vi "Stop case cleanup.vi"(11 "Next State":T1) -> ()   [LabVIEW 2013]
uses:
  Typedefs/Top level VI states.ctl
  Typedefs/Next state queue data.ctl
  Typedefs/Start-Stop Enum.ctl
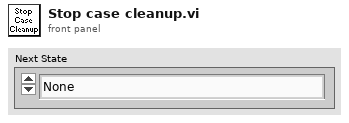
[diagram p1: front panel]
types:
  T1 = typedef "Top level VI states.ctl" = enum16{"None", "Initialise UI", "<STACK PROTOCOL STATES>", "AOL Zstack-START", "AOL Zstack-STOP", "Motor Zstack-START", "Motor Zstack-STOP", "<ACQUISITION PROTOCOL STATES> ", "Functional Acquisition-START", "Functional Acquisition-STOP", "Single Plane Acquisition-START", "Single Plane Acquisition-STOP", "Volume Acquisition-START", "Volume Acquisition-STOP", "<LIVE IMAGING PROTOCOL STATES>", "Live Imaging-START", "Live Imaging-STOP", "Live Plane Imaging-START", "Live Plane Imaging-STOP", "Live Volume Imaging-START", "Live Volume Imaging-STOP", "EXIT"}
  T2 = typedef "Start-Stop Enum.ctl" = enum16{"START", "STOP"}
  T3 = typedef "Next state queue data.ctl" = cluster{"Start/Stop":T2, "State":T1}
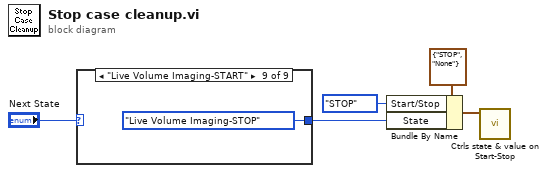
[diagram p0: block diagram]
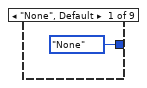
[diagram p2: hidden frame]
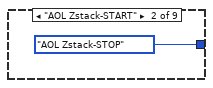
[diagram p3: hidden frame]
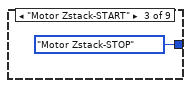
[diagram p4: hidden frame]
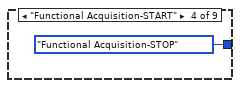
[diagram p5: hidden frame]
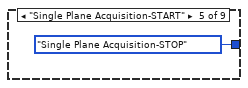
[diagram p6: hidden frame]
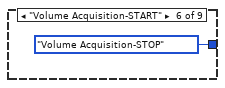
[diagram p7: hidden frame]
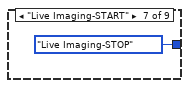
[diagram p8: hidden frame]
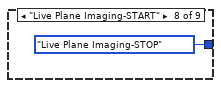
[diagram p9: hidden frame]
diagram:
  n1 = case shown="\"Live Volume Imaging-START\"" "Next State" {
    tunnel: [Top_level_VI_states."None" ("State") Top_level_VI_states."AOL Zstack-STOP" ("State") Top_level_VI_states."Motor Zstack-STOP" ("State") Top_level_VI_states."Functional Acquisition-STOP" ("State") Top_level_VI_states."Single Plane Acquisition-STOP" ("State") Top_level_VI_states."Volume Acquisition-STOP" ("State") Top_level_VI_states."Live Imaging-STOP" ("State") Top_level_VI_states."Live Plane Imaging-STOP" ("State") Top_level_VI_states."Live Volume Imaging-STOP" ("State")] -> w5
    frame "None", Default {
    }
    frame "AOL Zstack-START" {
    }
    frame "Motor Zstack-START" {
    }
    frame "Functional Acquisition-START" {
    }
    frame "Single Plane Acquisition-START" {
    }
    frame "Volume Acquisition-START" {
    }
    frame "Live Imaging-START" {
    }
    frame "Live Plane Imaging-START" {
    }
    frame "Live Volume Imaging-START" {
    }
  }
  n2 = Bundle By Name(cluster=T3 {"Start/Stop"=enum."STOP", "State"=enum."None"} ("Queue data"), "Start/Stop"=Start-Stop_Enum."STOP", "State"=w5) -> (w3:T3)
  n3 = call "Ctrls state & value on Start-Stop.vi"("Queue data"=w3) -> ()  [unwired: 10 in, 1 out]
